vi "Main.vi"(11 "Module Admin":refnum<class "Delacor_lib_QMH_Module Admin.lvclass">) -> ()   [LabVIEW 2025, in "Autofrettage UI.lvlib"]
doc: "This template is based off of the Queued Message Handler design pattern and the Queued Message Handler project template that ships with LabVIEW.\n\nThe main difference is that the queue is private to this module and communication between modules is performed via Broadcast and Request events.\n\nRequest events are wrapped in public API methods and are handled in the Event Handling Loop (EHL) of this VI. Any module can register for Broadcast events sent by this module. The EHL generates messages based on user interface actions.\n\nThe Message Handling Loop (MHL) processes messages generated by the EHL, or by other messages. The messages are string values, so new messages can be added easily to the Message Cases case structure in the MHL. Each message cluster can also provide an optional value for Message Data, which is a variant that can be converted to whatever message-specific data is required.\n_____\nBased on DQMH Project Template 4.0.0.47.\n_____\nBased on DQMH Dev Tools: Project Template 7.1.0.1503."
uses:
  Autofrettage UI.lvlib
  Module Data--cluster.ctl
  <vilib>/Delacor/Delacor QMH/Libraries/Message Queue_class/Delacor_lib_QMH_Message Queue.lvclass
  <vilib>/Delacor/Delacor QMH/Libraries/Message Queue_class/Delacor_lib_QMH_Enqueue Message (Single).vi
  <vilib>/Delacor/Delacor QMH/Libraries/Module Admin_class/Delacor_lib_QMH_Module Admin.lvclass
  Stop Argument--cluster.ctl
  Settings Editor/Settings Editor.lvlib
  Acquisition/Acquisition.lvlib
  Logger/Logger.lvlib
  Settings Editor/Test Meta Data.ctl
panel:
  out "Horizontal Pointer Slide":dbl(slide) scale=0.0..100000.0
  in  "Part Number":string
  in  "Job Number":string
  in  "Operator":string
  in  "ZERO":bool
  out "Numeric":dbl format="%.0f PSI"
  out "Data":waveform(dbl)[](graph)
  in  "Start Logging":bool
  in  "Settings":bool
  in  "Start":bool
  in  "Stop":bool
  out "error out":errorcluster
  out "Status":string
  in  "About":bool
  out "Logger Running?":bool
  out "Settings Editor Running?":bool
  out "Acquisition Running?":bool
  out "version":string
  # "Autofrettage"
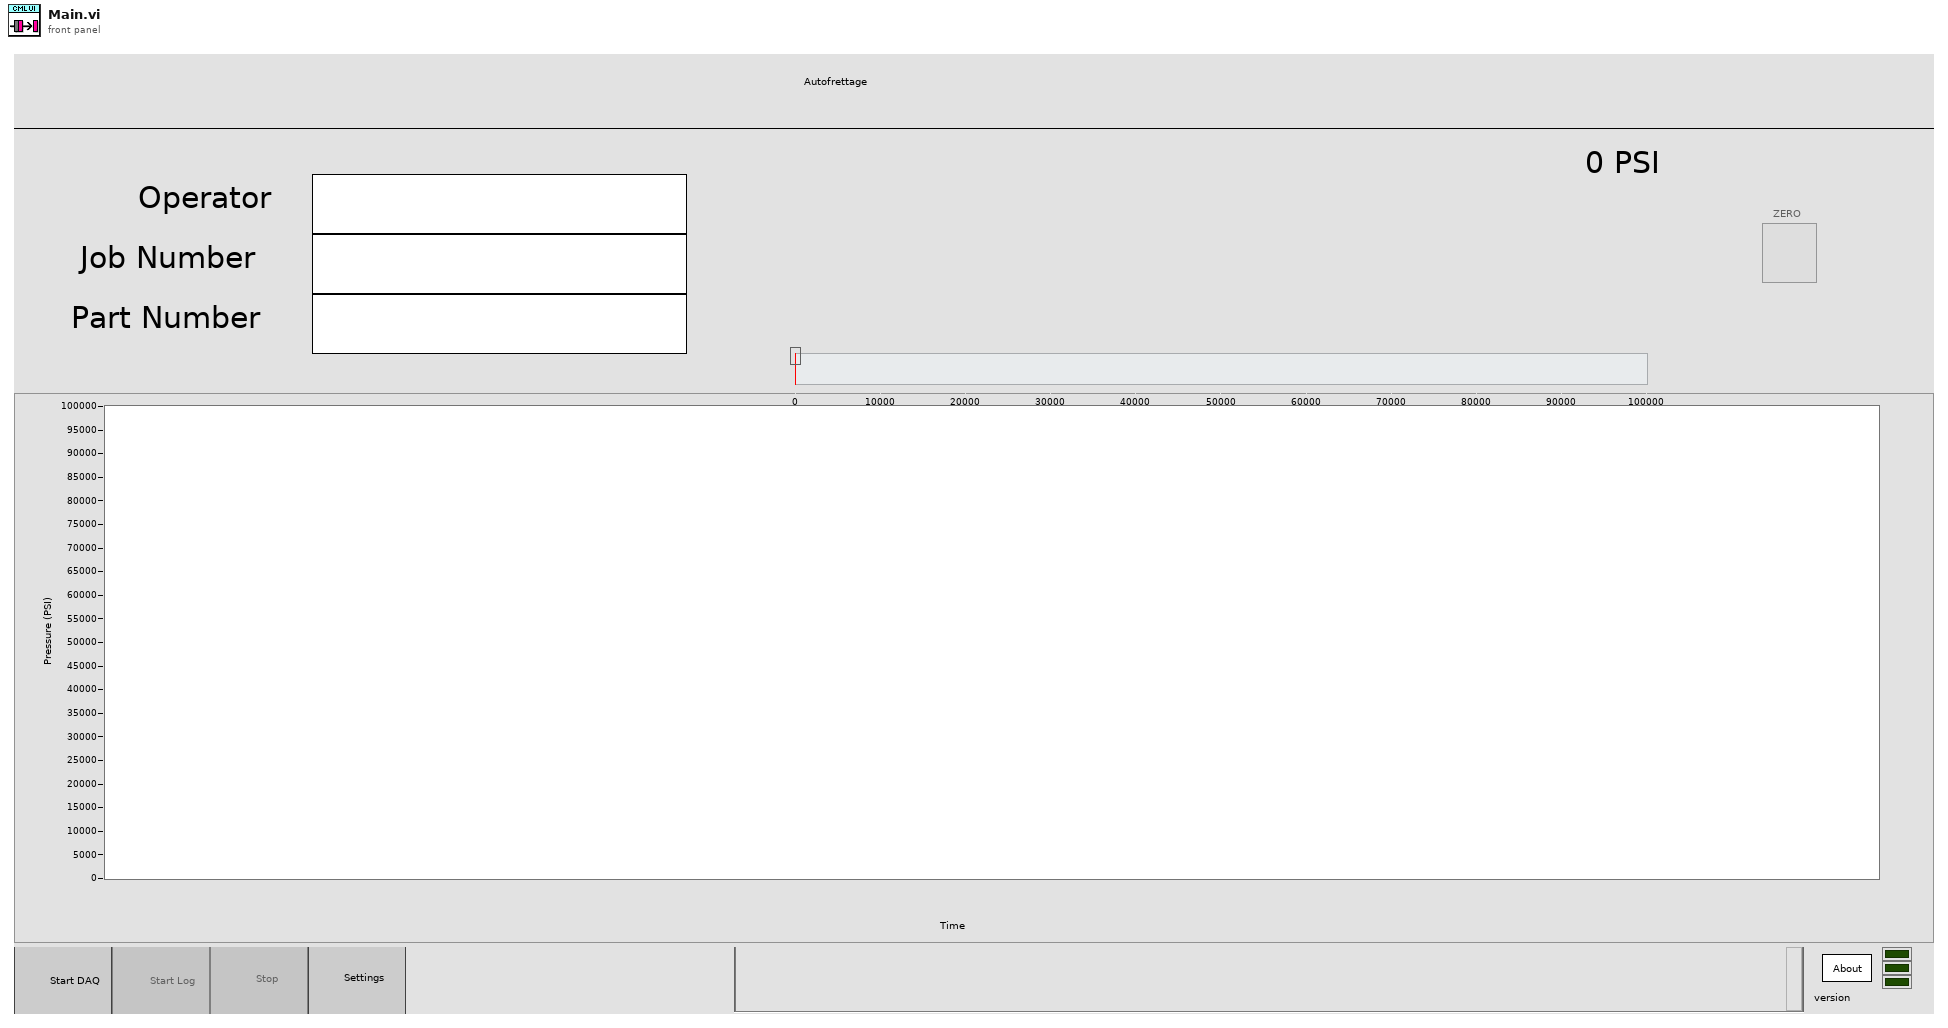
[diagram p1: front panel]
types:
  T1 = typedef "Autofrettage UI.lvlib/Request Events--cluster.ctl" = cluster{"Stop Module":refnum<user-event>, "Show Panel":refnum<user-event>, "Hide Panel":refnum<user-event>, "Get Module Execution Status":refnum<user-event>, "Show Diagram":refnum<user-event>}
  T2 = typedef "Settings Editor.lvlib/Broadcast Events--cluster.ctl" = cluster{"Module Did Init":refnum<user-event>, "Status Updated":refnum<user-event>, "Error Reported":refnum<user-event>, "Module Did Stop":refnum<user-event>, "Update Module Execution Status":refnum<user-event>, "Application Settings Updated":refnum<user-event>}
  T3 = typedef "Acquisition.lvlib/Broadcast Events--cluster.ctl" = cluster{"Module Did Init":refnum<user-event>, "Status Updated":refnum<user-event>, "Error Reported":refnum<user-event>, "Module Did Stop":refnum<user-event>, "Update Module Execution Status":refnum<user-event>, "Acquisition Started":refnum<user-event>, "Acquisition Stopped":refnum<user-event>, "Data Updated":refnum<user-event>, "Tare Updated":refnum<user-event>}
  T4 = typedef "Logger.lvlib/Broadcast Events--cluster.ctl" = cluster{"Module Did Init":refnum<user-event>, "Status Updated":refnum<user-event>, "Error Reported":refnum<user-event>, "Module Did Stop":refnum<user-event>, "Update Module Execution Status":refnum<user-event>, "Logging Stopped":refnum<user-event>, "File Initialized":refnum<user-event>}
  T5 = typedef "Autofrettage UI.lvlib/Module Data--cluster.ctl" = cluster{"Status":string, "Start DAQ Ref":refnum<vi>, "Settings Ref":refnum<vi>, "Stop Ref":refnum<vi>, "Status Ref":refnum<vi>, "Data Ref":refnum<vi>, "Start Logging Ref":refnum<vi>, "Tare Ref":refnum<vi>}
  T6 = enum32{"invalid lock state", "Not Locked", "Locked (No Password)", "Password-protected"}
  T7 = typedef "Autofrettage UI.lvlib/Stop Argument--cluster.ctl" = cluster{"Origin":string, "Exit via Stop Module Req?":bool, "Wait for Module to stop?":bool}
  T8 = enum32{"Invalid", "Standard", "Closed", "Hidden", "Minimized", "Maximized"}
  T9 = typedef "Settings Editor.lvlib/Test Meta Data.ctl" = cluster{"Operator":string, "Job Number":string, "Part Number":string}
  T10 = typedef "Settings Editor.lvlib/Update Application Settings (Reply Payload)--cluster.ctl" = cluster{"Settings":T11, "error":errorcluster}
  T11 = typedef "Settings Editor.lvlib/Settings--cluster.ctl" = cluster{"Log File Base Path":path, "Meta Data":T12, "DAQ Settings":cluster{"physical channel":string, "minimum value":dbl, "maximum value":dbl, "number of samples":i32, "rate":dbl, "custom scale name":string}}
  T12 = typedef "Test Meta Data.ctl" = cluster{"Operator":string, "Job Number":string, "Part Number":string}
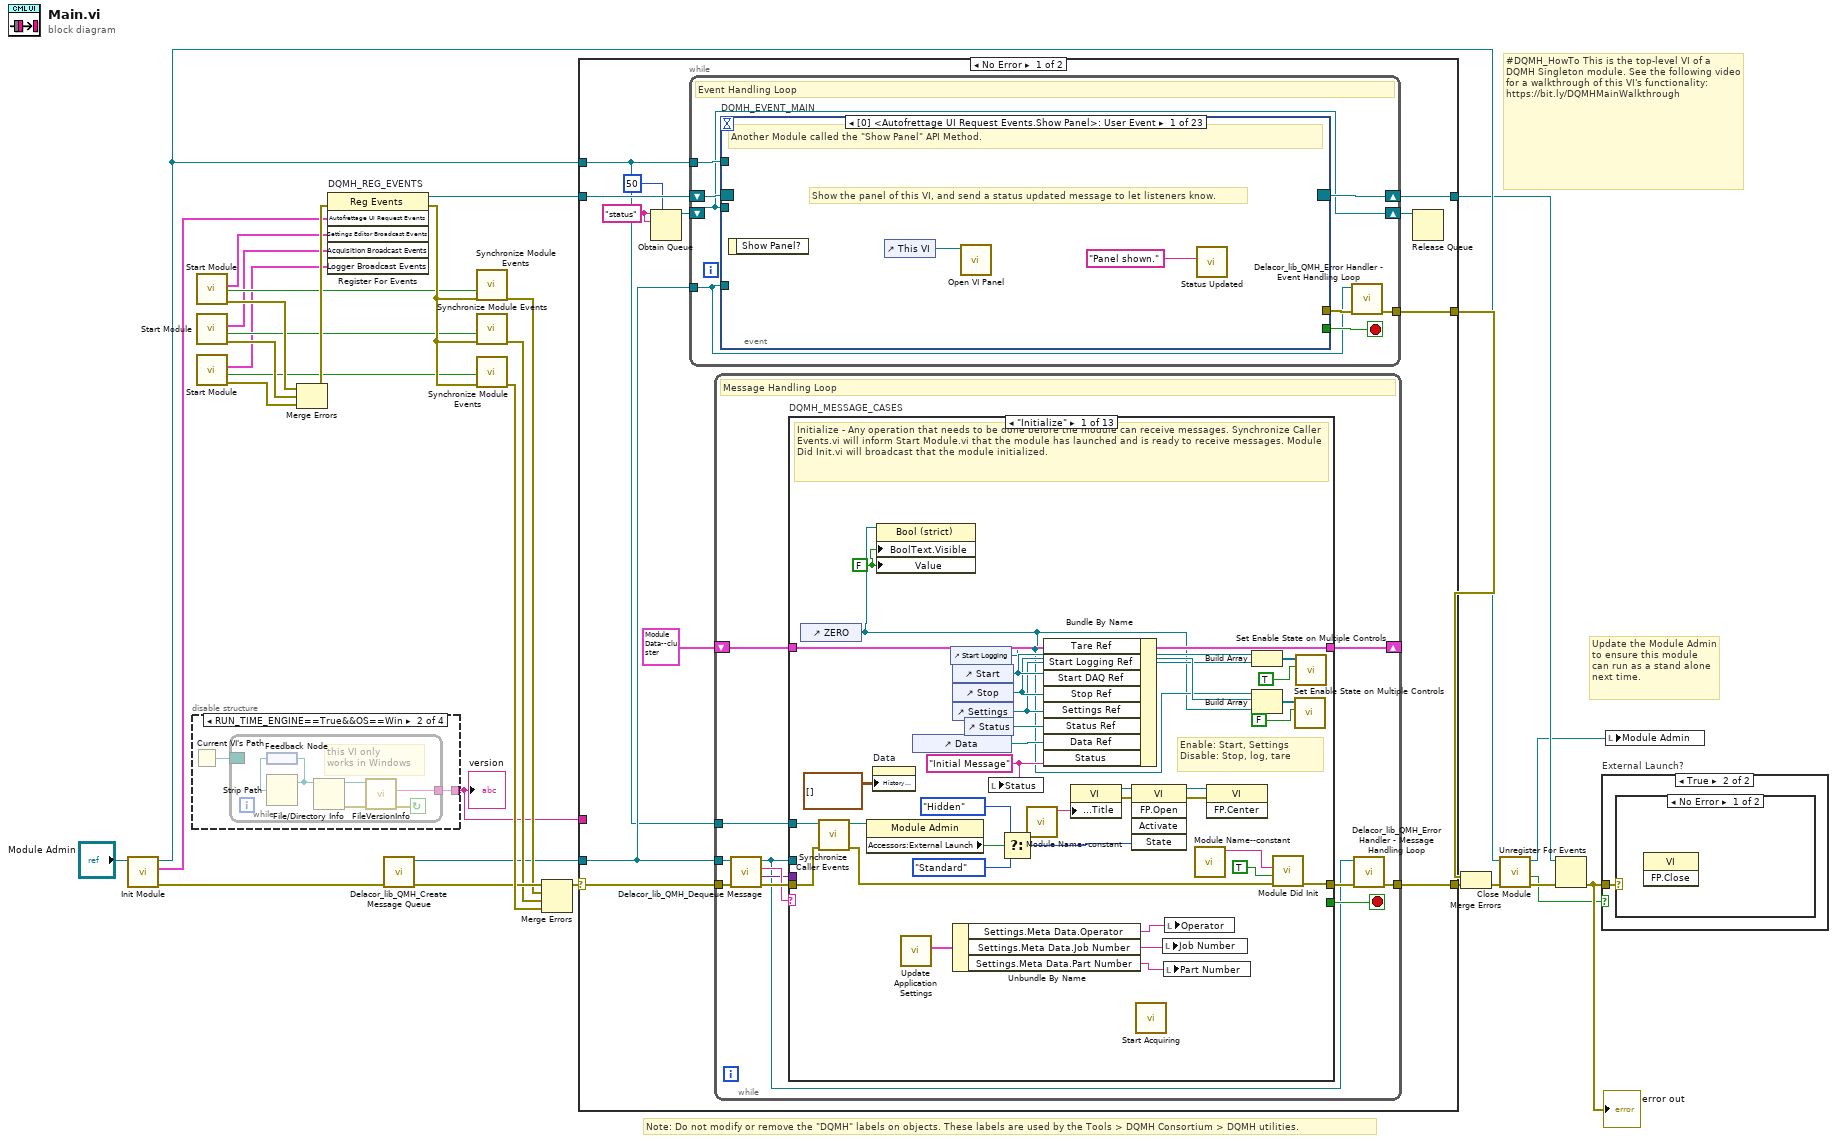
[diagram p0: block diagram]
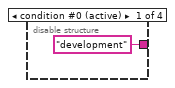
[diagram p2: hidden frame]
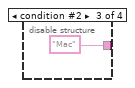
[diagram p3: hidden frame]
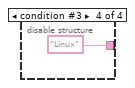
[diagram p4: hidden frame]
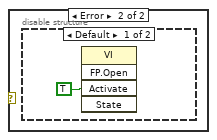
[diagram p6: hidden frame]
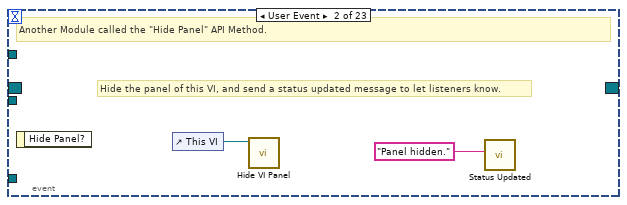
[diagram p8: hidden frame]
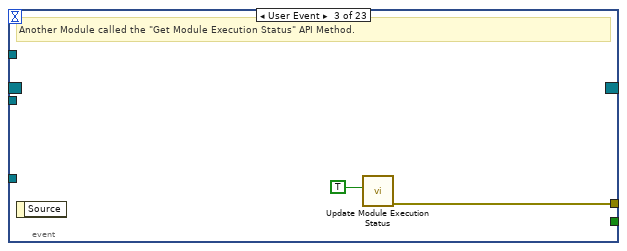
[diagram p9: hidden frame]
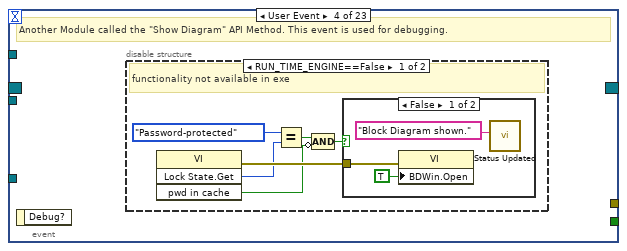
[diagram p10: hidden frame]
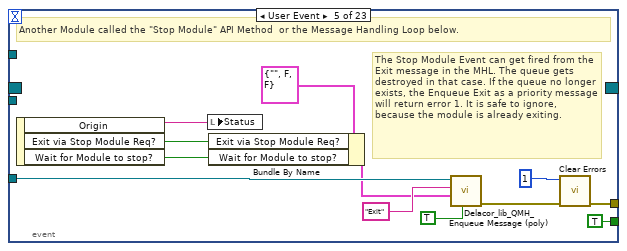
[diagram p13: hidden frame]
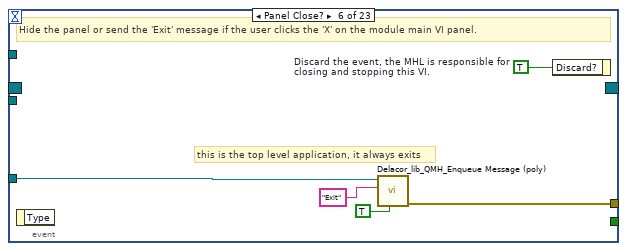
[diagram p14: hidden frame]
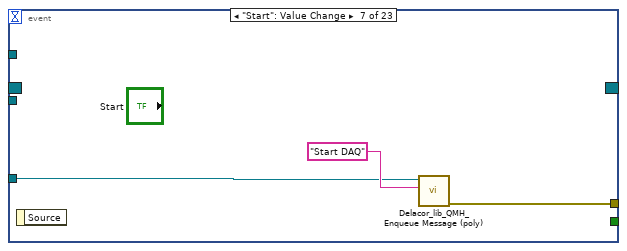
[diagram p15: hidden frame]
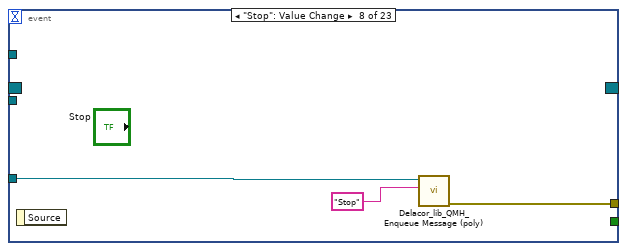
[diagram p16: hidden frame]
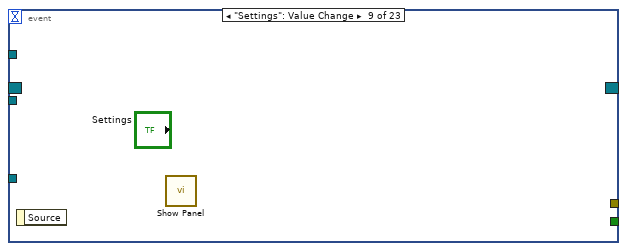
[diagram p17: hidden frame]
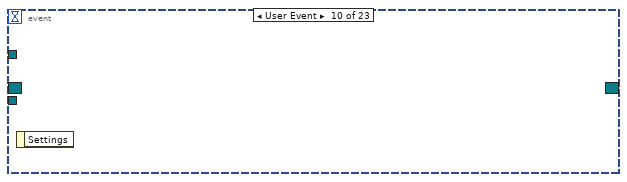
[diagram p18: hidden frame]
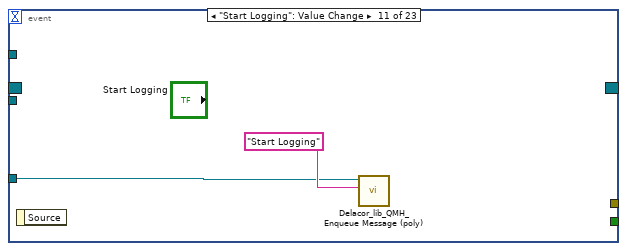
[diagram p19: hidden frame]
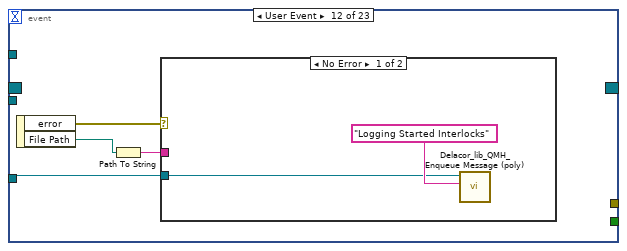
[diagram p20: hidden frame]
diagram:
  # "#DQMH_HowTo This is the top-level VI of a DQMH Singleton module. See the following video for a walkthrough of this VI's functionality: https://bit.ly/DQMHMainWalkthrough"
  # "Note: Do not modify or remove the \"DQMH\" labels on objects. These labels are used by the Tools > DQMH Consortium > DQMH utilities."
  # "Update the Module Admin to ensure this module can run as a stand alone next time."
  n1 = call "Init Module.vi"("Singleton Module Admin in"="Module Admin") -> ("error out"=w29:errorcluster, "Autofrettage UI Request Events"=w12:T1, "Singleton Module Admin out"=w15:refnum<class "Delacor_lib_QMH_Module Admin.lvclass">)  [unwired: 8 in]
  n2 = disable-structure "Conditional Disable Structure" shown="RUN_TIME_ENGINE==True&&OS==Win" {
    disable-tunnel: ["development" w33 "Mac" "Linux"] -> w1
    frame condition #0 (active) {
    }
    frame condition #1 {
      n3 = Current VI's Path() -> (path=w34:path)
      n4 = while {
        border: w34 -> [_]
        tunnel: [w35] -> w33
        stop <- w39 continue-if-true
        # "this VI only \nworks in Windows"
        n5 = feedback #1() -> (w38:path)
        n6 = Strip Path(path=w38) -> (stripped path=w37:path)  [unwired: 1 out]
        n7 = feedback-in #1(w37) -> ()
        n8 = File/Directory Info(path=w37) -> (path out=w36:path, error out=w40:errorcluster)  [unwired: 1 in, 5 out]
        n9 = call <vilib>:"FileVersionInfo.vi"("error in (no error)"=w40, "Application Path in"=w36) -> ("error out"=w39:errorcluster, "File Version Info"=w35:string)  [unwired: 6 in, 2 out]
      }
    }
    frame condition #2 {
    }
    frame condition #3 {
    }
  }
  "version" <- w1
  n10 = call "Start Module.vi"() -> ("error out"=w20:errorcluster, "Wait for Event Sync?"=w7:bool, "Settings Editor Broadcast Events"=w6:T2)  [unwired: 7 in, 2 out]
  n11 = call "Start Module.vi"() -> ("error out"=w19:errorcluster, "Wait for Event Sync?"=w4:bool, "Acquisition Broadcast Events"=w5:T3)  [unwired: 7 in, 2 out]
  n12 = call "Start Module.vi"() -> ("error out"=w18:errorcluster, "Wait for Event Sync?"=w2:bool, "Logger Broadcast Events"=w3:T4)  [unwired: 7 in, 2 out]
  n13 = Merge Errors(w20, w19, w18) -> (w17:errorcluster)
  n14 = register-events "DQMH_REG_EVENTS"(error in=w17, w12, w6, w5, w3) -> (reference out=w13:refnum<event-registration>, error out=w16:errorcluster)  [unwired: 1 in]
  n15 = call <vilib>:"Delacor_lib_QMH_Create Message Queue.vi"("error in"=w29) -> ("error out"=w24:errorcluster, "Message Queue"=w11:refnum<class "Delacor_lib_QMH_Message Queue.lvclass">)  [unwired: 9 in]
  n16 = call "Synchronize Module Events.vi"("error in"=w16, "Wait for Event Sync?"=w7) -> ("error out"=w22:errorcluster)  [unwired: 9 in]
  n17 = call "Synchronize Module Events.vi"("error in"=w16, "Wait for Event Sync?"=w4) -> ("error out"=w21:errorcluster)  [unwired: 9 in]
  n18 = call "Synchronize Module Events.vi"("error in"=w16, "Wait for Event Sync?"=w2) -> ("error out"=w31:errorcluster)  [unwired: 9 in]
  n19 = Merge Errors(w24, w22, w21, w31) -> (w23:errorcluster)
  n20 = case shown="No Error" w23 {
    selector: w23 -> [w52 w315]
    tunnel: [w54 w314] -> w30
    tunnel: [w51 w313] -> w14
    tunnel: w13 -> [w49 w313]
    tunnel: w11 -> [w48 w306]
    tunnel: [w53 _] -> w27
    tunnel: w15 -> [w47 w309]
    tunnel: w1 -> [_ _]
    frame No Error {
      w43 = "status" ("name (unnamed)")
      n21 = Obtain Queue(max queue size (-1, unlimited)=50, name (unnamed)=w43, element data type=w43) -> (queue out=w45:refnum<queue>)  [unwired: 2 in, 2 out]
      n22 = while {
        tunnel: w48 -> [w56]
        shift-right: [w59] -> w51
        shift-left: w49 -> [w60]
        tunnel: [w61] -> w53
        tunnel: w47 -> [w57]
        shift-right: [w55] -> w44
        shift-left: w45 -> [w55]
        stop <- w58 stop-if-true
        # "Event Handling Loop"
        n23 = event "DQMH_EVENT_MAIN" shown="[0] <Autofrettage UI Request Events.Show Panel>: User Event" {
          selector: w60 -> [_ _ _ _ _ _ _ _ _ _ _ _ _ _ w118 _ _ _ _ _ _ _ _]
          dyn-events: [_ _ _ _ _ _ _ _ _ _ _ _ _ _ w118 _ _ _ _ _ _ _ _] -> w59
          timeout: _ -> [_ _ _ _ _ _ _ _ _ _ _ _ _ _ _ _ _ _ _ _ _ _ _]
          tunnel: [_ _ _ _ TRUE ("Discard?") _ _ _ _ _ _ _ _ _ _ _ _ _ _ _ _ _ _] -> w58
          tunnel: w56 -> [_ _ _ _ w85 w92 w95 w98 _ _ w101 w103 _ _ _ _ _ _ w144 w148 _ _ _]
          tunnel: [_ _ w68 _ w88 w94 w97 w100 _ _ _ _ _ _ _ _ _ w139 _ _ _ _ w155] -> w62
          tunnel: w57 -> [_ _ _ _ _ _ _ _ _ _ _ _ _ _ _ _ _ _ _ _ _ _ _]
          tunnel: w55 -> [_ _ _ _ _ _ _ _ _ _ _ _ _ _ _ _ w133 _ _ _ _ _ _]
          event User Event {
            # "Show the panel of this VI, and send a status updated message to let listeners know."
            # "Another Module called the \"Show Panel\" API Method."
            n24 = event-data() -> ()  [unwired: 1 in, 1 out]
            n25 = control-ref of="This VI"() -> (w64:refnum<vi>)
            n26 = call "Open VI Panel.vi"("VI"=w64) -> ()  [unwired: 10 in, 1 out]
            n27 = call "Status Updated.vi"("Status"="Panel shown." ("format string")) -> ()  [unwired: 10 in, 1 out]
          }
          event User Event {
            # "Hide the panel of this VI, and send a status updated message to let listeners know."
            # "Another Module called the \"Hide Panel\" API Method."
            n28 = event-data() -> ()  [unwired: 1 in, 1 out]
            n29 = control-ref of="This VI"() -> (w66:refnum<vi>)
            n30 = call "Hide VI Panel.vi"("VI"=w66) -> ()  [unwired: 10 in, 1 out]
            n31 = call "Status Updated.vi"("Status"="Panel hidden." ("format string")) -> ()  [unwired: 10 in, 1 out]
          }
          event User Event {
            # "Another Module called the \"Get Module Execution Status\" API Method."
            n32 = event-data() -> ()  [unwired: 1 in, 1 out]
            n33 = call "Update Module Execution Status.vi"("Running?"=TRUE) -> ("error out"=w68:errorcluster)  [unwired: 10 in]
          }
          event User Event {
            # "Another Module called the \"Show Diagram\" API Method. This event is used for debugging."
            n34 = event-data() -> ()  [unwired: 1 in, 1 out]
            n35 = disable-structure shown="RUN_TIME_ENGINE==False" {
              frame condition #0 (active) {
                # "functionality not available in exe"
                n36 = invoke on="Invoke Node" class="VI" method="Lock State.Get"() -> (error out=w74:errorcluster, "Get Lock State"=w73:T6, "pwd in cache"=w70:bool)  [unwired: 4 in, 1 out]
                n37 = Equal?(x=T6."Password-protected", y=w73) -> (x = y?=w71:bool)
                n38 = Compound Arithmetic op=AND(w71, invert w70) -> (w69:bool)
                n39 = case shown="False" w69 {
                  tunnel: w74 -> [w77 _]
                  frame False {
                    n40 = property on="Property Node" class="VI"(error in=w77, "BDWin.Open"=TRUE ("Block Diagram Window:Open")) -> ()  [unwired: 1 in, 2 out]
                    n41 = call "Status Updated.vi"("Status"="Block Diagram shown." ("format string")) -> ()  [unwired: 10 in, 1 out]
                  }
                  frame True {
                    # "Password-protected VI, and the password is not in the cache. Do not show the diagram."
                  }
                }
              }
              frame condition #1 {
              }
            }
          }
          event User Event {
            # "The Stop Module Event can get fired from the Exit message in the MHL. The queue gets destroyed in that case. If the queue no longer exists, the Enqueue Exit as a priority message will return error 1. It is safe to ignore, because the module is already exiting."
            # "Another Module called the \"Stop Module\" API Method  or the Message Handling Loop below."
            n42 = event-data() -> ("Origin"=w84:string, "Exit via Stop Module Req?"=w80:bool, "Wait for Module to stop?"=w79:bool)  [unwired: 1 in]
            n43 = local write "Status"(w84) -> ()
            n44 = Bundle By Name(cluster=T7 {"Origin"="", "Exit via Stop Module Req?"=FALSE, "Wait for Module to stop?"=FALSE} ("Stop Argument"), "Exit via Stop Module Req?"=w80, "Wait for Module to stop?"=w79) -> (w78:T7)
            n45 = call-poly <vilib>:"Delacor_lib_QMH_Enqueue Message (poly).vi"("Priority Message? (F)"=TRUE, "Message Data"=w78, "Message"="Exit", "Message Queue in"=w85) -> ("error out"=w89:errorcluster)  [unwired: 6 in, 1 out]
            n46 = call <vilib>:"Clear Errors.vi"("error in (no error)"=w89, "specific error code to clear (0: all)"=1) -> ("error out"=w88:errorcluster)  [unwired: 4 in, 1 out]
          }
          event Panel Close? {
            w93 = TRUE  # Discard the event, the MHL is responsible for closing and stopping this VI.
            # "this is the top level application, it always exits"
            # "Hide the panel or send the 'Exit' message if the user clicks the 'X' on the module main VI panel."
            n47 = event-data() -> ()  [unwired: 1 in, 1 out]
            n48 = call-poly <vilib>:"Delacor_lib_QMH_Enqueue Message (poly).vi"("Priority Message? (F)"=TRUE, "Message"="Exit", "Message Queue in"=w92) -> ("error out"=w94:errorcluster)  [unwired: 7 in, 1 out]
            n49 = event-data ("Event Filter Node")("Discard?"=w93) -> ()  [unwired: 1 in, 1 out]
          }
          event "Start": Value Change {
            n50 = event-data() -> ()  [unwired: 1 in, 1 out]
            n51 = call-poly <vilib>:"Delacor_lib_QMH_Enqueue Message (poly).vi"("Message"="Start DAQ", "Message Queue in"=w95) -> ("error out"=w97:errorcluster)  [unwired: 8 in, 1 out]
          }
          event "Stop": Value Change {
            n52 = event-data() -> ()  [unwired: 1 in, 1 out]
            n53 = call-poly <vilib>:"Delacor_lib_QMH_Enqueue Message (poly).vi"("Message"="Stop", "Message Queue in"=w98) -> ("error out"=w100:errorcluster)  [unwired: 8 in, 1 out]
          }
          event "Settings": Value Change {
            n54 = event-data() -> ()  [unwired: 1 in, 1 out]
            n55 = call "Show Panel.vi"() -> ()  [unwired: 11 in, 1 out]
          }
          event User Event {
            n56 = event-data() -> ()  [unwired: 1 in, 1 out]
          }
          event "Start Logging": Value Change {
            n57 = event-data() -> ()  [unwired: 1 in, 1 out]
            n58 = call-poly <vilib>:"Delacor_lib_QMH_Enqueue Message (poly).vi"("Message"="Start Logging", "Message Queue in"=w101) -> ()  [unwired: 8 in, 2 out]
          }
          event User Event {
            n59 = event-data() -> ("error"=w106:errorcluster, "File Path"=w105:path)  [unwired: 1 in]
            n60 = Path To String(path=w105) -> (string=w104:string)
            n61 = case shown="No Error" w106 {
              tunnel: w104 -> [_ _]
              tunnel: w103 -> [w107 _]
              frame No Error {
                n62 = call-poly <vilib>:"Delacor_lib_QMH_Enqueue Message (poly).vi"("Message"="Logging Started Interlocks", "Message Queue in"=w107) -> ()  [unwired: 8 in, 2 out]
              }
              frame Error {
              }
            }
          }
          event "ZERO": Value Change {
            n63 = event-data() -> ()  [unwired: 1 in, 1 out]
            n64 = call "Set Tare.vi"("Tare"="ZERO") -> ()  [unwired: 10 in, 1 out]
          }
          event User Event {
            w111 = TRUE ("Settings Editor Running?")
            n65 = event-data() -> ()  [unwired: 1 in, 1 out]
            n66 = local read "Acquisition Running?"() -> (w113:bool)
            n67 = local read "Logger Running?"() -> (w112:bool)
            n68 = call "Is UI Ready.vi"("Logger Running?"=w112, "Acquisition Running?"=w113, "Settings Editor Running?"=w111) -> ("Status"=w110:string)  [unwired: 8 in]
            n69 = local write "Status"(w110) -> ()
            "Settings Editor Running?" <- w111
          }
          event User Event {
            w116 = TRUE ("Acquisition Running?")
            n70 = event-data() -> ()  [unwired: 1 in, 1 out]
            n71 = local read "Settings Editor Running?"() -> (w115:bool)
            n72 = local read "Logger Running?"() -> (w114:bool)
            n73 = call "Is UI Ready.vi"("Logger Running?"=w114, "Acquisition Running?"=w116, "Settings Editor Running?"=w115) -> ("Status"=w117:string)  [unwired: 8 in]
            n74 = local write "Status"(w117) -> ()
            "Acquisition Running?" <- w116
          }
          event User Event {
            w121 = TRUE ("Logger Running?")
            n75 = event-data() -> ()  [unwired: 1 in, 1 out]
            n76 = local read "Settings Editor Running?"() -> (w120:bool)
            n77 = local read "Acquisition Running?"() -> (w119:bool)
            n78 = call "Is UI Ready.vi"("Logger Running?"=w121, "Acquisition Running?"=w119, "Settings Editor Running?"=w120) -> ("Status"=w122:string)  [unwired: 8 in]
            n79 = local write "Status"(w122) -> ()
            "Logger Running?" <- w121
          }
          event User Event {
            n80 = event-data() -> ("Status"=w125:string)  [unwired: 1 in]
            n81 = Format Date/Time String(time format string (%c)="%H:%M:%S%3u") -> (date/time string=w127:string)  [unwired: 2 in]
            n82 = Format Into String(format string="%s: %s", w127, w125) -> (resulting string=w124:string)  [unwired: 2 in, 1 out]
            n83 = Lossy Enqueue Element(queue=w133, element=w124) -> (queue out=w132:refnum<queue>)  [unwired: 1 in, 3 out]
            n84 = Get Queue Status(queue=w132, return elements? (F)=TRUE) -> (elements=w130:string[])  [unwired: 1 in, 7 out]
            n85 = Reverse 1D Array(array=w130) -> (reversed array=w129:string[])
            n86 = for {
              tunnel: w129 -> [w136] mode=indexing
              tunnel: [w134] -> w128 mode=concatenating
              n87 = Concatenate Strings(w136, "\r\n") -> (w134:string)
            }
            "Status" <- w128
            n88 = call "Status Updated.vi"("Status"=w128) -> ()  [unwired: 10 in, 1 out]
          }
          event User Event {
            n89 = event-data() -> ("Error"=w139:errorcluster, "Module Name"=w141:string)  [unwired: 1 in]
            n90 = Unbundle By Name(w139) -> ("code"=w142:i32)
            n91 = Format Into String(format string="Error %d at %s", w142, w141) -> (resulting string=w138:string)  [unwired: 2 in, 1 out]
            n92 = Bundle By Name(cluster=w139, "source"=w138) -> (w137:errorcluster)
            n93 = call <vilib>:"Simple Error Handler.vi"("error in (no error)"=w137) -> ()  [unwired: 4 in, 5 out]
          }
          event User Event {
            n94 = event-data() -> ("Success"=w143:bool)  [unwired: 1 in]
            n95 = case shown="True" w143 {
              tunnel: w144 -> [_ w146]
              frame False {
              }
              frame True {
                n96 = call-poly <vilib>:"Delacor_lib_QMH_Enqueue Message (poly).vi"("Message"="Acquisition Started Interlocks", "Message Queue in"=w146) -> ()  [unwired: 8 in, 2 out]
              }
            }
          }
          event User Event {
            n97 = event-data() -> ()  [unwired: 1 in, 1 out]
            n98 = call-poly <vilib>:"Delacor_lib_QMH_Enqueue Message (poly).vi"("Message"="Acquisition Stopped Interlocks", "Message Queue in"=w148) -> ()  [unwired: 8 in, 2 out]
          }
          event User Event {
            n99 = event-data() -> ("Numeric"=→"Numeric" →"Horizontal Pointer Slide":dbl, "Graph Data"=→"Data":waveform(dbl)[])  [unwired: 1 in]
          }
          event User Event {
            n100 = event-data() -> ("Tare Offset"=w154:dbl)  [unwired: 1 in]
            n101 = Not Equal To 0?(x=w154) -> (x != 0?=w151:bool)
            n102 = Format Into String(format string="%d", w154) -> (resulting string=w152:string)  [unwired: 2 in, 1 out]
            n103 = property on="ZERO" class="Bool (strict)"("Value"=w151, "BoolText.Visible"=w151, "BoolText.Text"=w152) -> ()  [unwired: 2 in, 2 out]
          }
          event "About": Value Change {
            # "Display the About DQMH box"
            n104 = event-data() -> ()  [unwired: 1 in, 1 out]
            n105 = call <vilib>:"DQMH_About Box.vi"() -> ("error out"=w155:errorcluster)  [unwired: 11 in]
          }
        }
        n106 = call-dynamic "Delacor_lib_QMH_Error Handler - Event Handling Loop.vi"("error in"=w62, "Message Queue in"=w56) -> ("dup error in"=w61:errorcluster)  [unwired: 8 in, 1 out]
      }
      n107 = while {
        tunnel: w48 -> [w158]
        shift-right: [w162] -> _
        shift-left: T5 {"Status"="", "Start DAQ Ref"=refnum, "Settings Ref"=refnum, "Stop Ref"=refnum, "Status Ref"=refnum, "Data Ref"=refnum, "Start Logging Ref"=refnum, "Tare Ref"=refnum} ("Data Cluster") -> [w163]
        tunnel: w52 -> [w166]
        tunnel: [w164] -> w54
        tunnel: w47 -> [w156]
        stop <- w161 stop-if-true
        # "Message Handling Loop"
        n108 = call-dynamic "Delacor_lib_QMH_Dequeue Message.vi"("error in"=w166, "Message Queue in"=w158) -> ("error out"=w165:errorcluster, "Message Data"=w159:variant, "Message"=w160:string, "Message Queue out"=w157:refnum<class "Delacor_lib_QMH_Message Queue.lvclass">)  [unwired: 6 in]
        n109 = case "DQMH_MESSAGE_CASES" shown="\"Initialize\"" w160 {
          selector: w160 -> [_ _ _ _ _ _ _ _ _ _ _ _ w301]
          tunnel: w157 -> [_ _ _ _ _ _ _ _ _ _ w260 w285 _]
          tunnel: w165 -> [w201 w205 w206 w215 w231 w234 w247 w252 w255 w257 w268 w293 w304]
          tunnel: [w199 w205 w208 w216 w231 w233 w247 w252 w254 w257 w264 w286 w305] -> w167
          tunnel: w163 -> [w190 w204 w207 w217 w223 w232 w239 w249 w253 w256 w262 w284 w302]
          tunnel: [w182 w204 w207 w217 w223 w232 w239 w249 w253 w256 w262 w284 w302] -> w162
          tunnel: [_ _ _ _ _ _ _ _ _ _ _ w283 _] -> w161
          tunnel: w159 -> [_ _ _ _ _ _ _ _ _ _ w261 w282 _]
          tunnel: w156 -> [w191 _ _ _ _ _ _ _ _ _ w259 w277 _]
          frame "Initialize" {
            w169 = FALSE ("Value")
            w185 = "Initial Message" ("Initial Message")
            # "Enable: Start, Settings\nDisable: Stop, log, tare"
            # "Initialize - Any operation that needs to be done before the module can receive messages. Synchronize Caller Events.vi will inform Start Module.vi that the module has launched and is ready to receive messages. Module Did Init.vi will broadcast that the module initialized."
            n110 = control-ref of="ZERO"() -> (w168:refnum<vi>)
            n111 = call "Synchronize Caller Events.vi"("error in"=w201, "Singleton Module Admin in"=w191) -> ("error out"=w200:errorcluster, "Singleton Module Admin out"=w187:refnum<class "Delacor_lib_QMH_Module Admin.lvclass">)  [unwired: 8 in]
            n112 = property on="Property Node" class="Module Admin"(reference=w187) -> ("Accessors:External Launch"=w195:bool)  [unwired: 1 in, 2 out]
            n113 = property on="Data" class="WFChart (strict)"("History Data"=waveform(dbl)[][] []) -> ()  [unwired: 2 in, 2 out]
            n114 = property class="Bool (strict)"(reference=w168, "BoolText.Visible"=w169, "Value"=w169) -> ()  [unwired: 1 in, 2 out]
            n115 = call "Update Application Settings.vi"() -> ("Reply Payload"=w170:T10)  [unwired: 9 in, 2 out]
            n116 = control-ref of="Data"() -> (w183:refnum<vi>)
            n117 = control-ref of="Start Logging"() -> (w174:refnum<vi>)
            n118 = control-ref of="Start"() -> (w177:refnum<vi>)
            n119 = control-ref of="Stop"() -> (w176:refnum<vi>)
            n120 = control-ref of="Settings"() -> (w175:refnum<vi>)
            n121 = Unbundle By Name(w170) -> ("Settings.Meta Data.Operator"=w171:string, "Settings.Meta Data.Job Number"=w172:string, "Settings.Meta Data.Part Number"=w173:string)
            n122 = control-ref of="Status"() -> (w184:refnum<vi>)
            n123 = local write "Status"(w185) -> ()
            n124 = Select(t=T8."Hidden" ("State"), s=w195, f=T8."Standard" ("State")) -> (s? t:f=w192:T8)
            n125 = call "Module Name--constant.vi"() -> ("Module Name"=w198:string)  [unwired: 11 in]
            n126 = Bundle By Name(cluster=w190, "Tare Ref"=w168, "Start Logging Ref"=w174, "Start DAQ Ref"=w177, "Stop Ref"=w176, "Settings Ref"=w175, "Status Ref"=w184, "Data Ref"=w183, "Status"=w185) -> (w182:T5)
            n127 = property on="Property Node" class="VI"("Front Panel.Title"=w198) -> (reference out=w197:refnum<vi>, error out=w203:errorcluster)  [unwired: 2 in]
            n128 = invoke on="Invoke Node" class="VI" method="FP.Open"(reference=w197, error in=w203, "State"=w192) -> (reference out=w196:refnum<vi>, error out=w202:errorcluster)  [unwired: 2 in, 3 out]
            n129 = call "Start Acquiring.vi"() -> ()  [unwired: 9 in, 3 out]
            n130 = local write "Job Number"(w172) -> ()
            n131 = local write "Part Number"(w173) -> ()
            n132 = local write "Operator"(w171) -> ()
            n133 = call "Module Name--constant.vi"() -> ("Module Name"=w188:string)  [unwired: 11 in]
            n134 = invoke on="Invoke Node" class="VI" method="FP.Center"(reference=w196, error in=w202) -> ()  [unwired: 1 in, 3 out]
            n135 = Build Array(w177, w175) -> (w181:refnum<vi>[])
            n136 = Build Array(w174, w176, w168) -> (w179:refnum<vi>[])
            n137 = call "Module Did Init.vi"("error in"=w200, "Initialized?"=TRUE, "Origin"=w188) -> ("error out"=w199:errorcluster)  [unwired: 8 in]
            n138 = call "Set Enable State on Multiple Controls.vi"("Enable?"=FALSE, "Controls"=w179) -> ()  [unwired: 10 in]
            n139 = call "Set Enable State on Multiple Controls.vi"("Enable?"=TRUE, "Controls"=w181) -> ()  [unwired: 10 in]
          }
          frame "---Module Specific---" {
            # "Separator -- The following cases handle messages specific to this Module."
          }
          frame "Start DAQ" {
            # "End user pressed Start button. Need to request for Acquisition to start acquiring and for Logger to start logging."
            n140 = call "Start Acquiring.vi"("error in"=w206) -> ("error out"=w208:errorcluster)  [unwired: 8 in, 2 out]
          }
          frame "Start Logging" {
            # "End user pressed Start button. Need to request for Acquisition to start acquiring and for Logger to start logging."
            n141 = Bundle By Name(cluster=T9 {"Operator"="", "Job Number"="", "Part Number"=""} ("Test Meta Data"), "Operator"="Operator", "Job Number"="Job Number", "Part Number"="Part Number") -> (w212:T9)
            n142 = call "Save Test Meta Data.vi"("error in"=w215, "Test Meta Data"=w212) -> ("error out"=w214:errorcluster)  [unwired: 8 in, 1 out]
            n143 = case shown="No Error" w214 {
              selector: w214 -> [w218 w220]
              tunnel: [w219 w220] -> w216
              frame No Error {
                n144 = call "Initialize File.vi"("error in"=w218) -> ("error out"=w219:errorcluster)  [unwired: 8 in, 2 out]
              }
              frame Error {
              }
            }
          }
          frame "Acquisition Started Interlocks" {
            # "Enable: Stop\nDisable: Start, Settings"
            n145 = Unbundle By Name(w223) -> ("Tare Ref"=w221:refnum<vi>, "Start Logging Ref"=w222:refnum<vi>, "Stop Ref"=w230:refnum<vi>, "Start DAQ Ref"=w225:refnum<vi>, "Settings Ref"=w224:refnum<vi>)
            n146 = Build Array(w225, w224) -> (w226:refnum<vi>[])
            n147 = Build Array(w221, w230, w222) -> (w229:refnum<vi>[])
            n148 = call "Set Enable State on Multiple Controls.vi"("Enable?"=FALSE, "Controls"=w226) -> ()  [unwired: 10 in]
            n149 = call "Set Enable State on Multiple Controls.vi"("Enable?"=TRUE, "Controls"=w229) -> ()  [unwired: 10 in]
          }
          frame "Stop" {
            # "End user pressed Stop button. Need to request for Acquisition to stop acquiring and for Logger to stop logging."
            n150 = call "Stop Acquiring.vi"("error in"=w234) -> ("error out"=w235:errorcluster)  [unwired: 10 in]
            n151 = call "Stop Logging.vi"("error in"=w235) -> ("error out"=w233:errorcluster)  [unwired: 10 in]
          }
          frame "Acquisition Stopped Interlocks" {
            w237 = FALSE ("Value")
            # "Enable: Start, Settings\nDisable: Stop"
            n152 = Unbundle By Name(w239) -> ("Tare Ref"=w236:refnum<vi>, "Start Logging Ref"=w238:refnum<vi>, "Stop Ref"=w244:refnum<vi>, "Start DAQ Ref"=w243:refnum<vi>, "Settings Ref"=w242:refnum<vi>)
            n153 = Build Array(w243, w242) -> (w241:refnum<vi>[])
            n154 = Build Array(w236, w238, w244) -> (w246:refnum<vi>[])
            n155 = property class="Bool (strict)"(reference=w236, "BoolText.Visible"=w237, "Value"=w237) -> ()  [unwired: 1 in, 2 out]
            n156 = call "Set Enable State on Multiple Controls.vi"("Enable?"=TRUE, "Controls"=w241) -> ()  [unwired: 10 in]
            n157 = call "Set Enable State on Multiple Controls.vi"("Enable?"=FALSE, "Controls"=w246) -> ()  [unwired: 10 in]
          }
          frame "Logging Started Interlocks" {
            # "Enable: Start, Settings\nDisable: Stop"
            n158 = Unbundle By Name(w249) -> ("Start Logging Ref"=w248:refnum<vi>)
            n159 = Build Array(w248) -> (w251:refnum<vi>[])
            n160 = call "Set Enable State on Multiple Controls.vi"("Enable?"=FALSE, "Controls"=w251) -> ()  [unwired: 10 in]
          }
          frame "---Copy This Frame---" {
            # "Duplicate this frame when creating new messages.  Change this comment in the duplicated frame to describe this message."
            n161 = Merge Errors(w255) -> (w254:errorcluster)
          }
          frame "---Exit and Error Handling---" {
            # "Separator - The following cases handle errors and exit messages."
          }
          frame "Error" {
            # "Error - Check the error message data and respond accordingly. This message is sent by the \"Error Handler\" VIs at the end of each loop in this application."
            n162 = property on="Property Node" class="Module Admin"(reference=w259) -> ("Accessors:External Launch"=w258:bool)  [unwired: 1 in, 2 out]
            n163 = Variant To Data(error in=w268, type=errorcluster {"status"=FALSE, "code"=0, "source"=""} ("error constant"), Variant=w261) -> (data=w263:errorcluster, error out=w266:errorcluster)
            n164 = local write "error out"(w263) -> ()
            n165 = call "Error Reported.vi"("Error"=w263) -> ()  [unwired: 10 in, 1 out]
            n166 = case shown="False" w258 {
              tunnel: [w273 _] -> w265
              tunnel: w260 -> [w271 _]
              tunnel: w263 -> [w272 _]
              frame False {
                n167 = disable-structure shown="Default" {
                  disable-tunnel: w272 -> [w274 _]
                  frame condition #0 (active) {
                    # "If the module is running standalone, then pop up an error dialog and call the \"Exit\" message."
                    n168 = call <vilib>:"Simple Error Handler.vi"("error in (no error)"=w274) -> ()  [unwired: 4 in, 5 out]
                  }
                  frame condition #1 {
                    # "To prevent the Simple Error Handler VI from being loaded (e.g. when deploying to a Real-Time target), add the Conditional Disable Symbol \"DQMH_Disable_SEH\" to your project and set it to TRUE."
                  }
                }
                n169 = call-poly <vilib>:"Delacor_lib_QMH_Enqueue Message (poly).vi"("Priority Message? (F)"=TRUE, "Message"="Exit", "Message Queue in"=w271) -> ("error out"=w273:errorcluster)  [unwired: 7 in, 1 out]
              }
              frame True {
                # "If the module was launched externally, calling the Error Reported broadcast VI is the only action performed by the \"Error\" message. The module's caller can then process the error appropriately."
              }
            }
            n170 = Merge Errors(w266, w265) -> (w264:errorcluster)
          }
          frame "Exit" {
            w276 = TRUE ("Wait for Module to Stop? (F)")
            w283 = TRUE  # Stop the VI
            # "DAQ and LOG modules use the settings editor. CML UI module waits for both modules to completely stop before stopping the settings editor."
            # "Release the message queue reference"
            # "Exit - Exit the application."
            n171 = Variant To Data(error in=w293, type=T7 {"Origin"="", "Exit via Stop Module Req?"=FALSE, "Wait for Module to stop?"=FALSE} ("Stop Argument"), Variant=w282) -> (data=w279:T7, error out=w290:errorcluster)
            n172 = call <vilib>:"Clear Errors.vi"("error in (no error)"=w290, "specific error code to clear (0: all)"=91 ("91: not all Exit messages will have an argument")) -> ("error out"=w292:errorcluster)  [unwired: 4 in, 1 out]
            n173 = control-ref of="This VI"() -> (w278:refnum<vi>)
            n174 = call "Module Name--constant.vi"() -> ("Module Name"=w275:string)  [unwired: 11 in]
            n175 = call "Handle Exit.vi"("Stop Argument"=w279, "Admin in"=w277, "VI reference"=w278) -> ("error out"=w289:errorcluster)  [unwired: 7 in, 1 out]
            n176 = call "Stop Module.vi"("Wait for Module to Stop? (F)"=w276, "Origin"=w275) -> ("error out"=w288:errorcluster)  [unwired: 9 in]
            n177 = call "Stop Module.vi"("Wait for Module to Stop? (F)"=w276, "Origin"=w275) -> ("error out"=w287:errorcluster)  [unwired: 9 in]
            n178 = call-dynamic "Delacor_lib_QMH_Release Message Queue.vi"("error in"=w292, "Message Queue"=w285) -> ("error out"=w291:errorcluster)  [unwired: 9 in]
            n179 = Merge Errors(w288, w287) -> (w294:errorcluster)
            n180 = Merge Errors(w291, w289) -> (w286:errorcluster)
            n181 = call <vilib>:"Clear Errors.vi"("error in (no error)"=w294) -> ("error out"=w295:errorcluster)  [unwired: 5 in, 1 out]
            n182 = call "Error Reported.vi"("Error"=w286) -> ()  [unwired: 10 in, 1 out]
            n183 = call "Stop Module.vi"("error in"=w295, "Wait for Module to Stop? (F)"=w276, "Origin"=w275) -> ()  [unwired: 8 in, 1 out]
          }
          frame Default {
            # "'Default' case only runs if there is a message that isn't defined in any of the other cases.  Output a programming error."
            n184 = call "Module Name--constant.vi"() -> ("Module Name"=w300:string)  [unwired: 11 in]
            n185 = Format Into String(format string="The invalid message string \"%s\" was received in the Message Handling Loop for module \"%s\".", w301, w300) -> (resulting string=w298:string)  [unwired: 2 in, 1 out]
            n186 = call <vilib>:"Error Cluster From Error Code.vi"("show call chain? (False)"=TRUE, "error message (\"\")"=w298, "error code (0)"=1) -> ("error out"=w303:errorcluster)  [unwired: 6 in]
            n187 = Merge Errors(w304, w303) -> (w305:errorcluster)
          }
        }
        n188 = call-dynamic "Delacor_lib_QMH_Error Handler - Message Handling Loop.vi"("error in"=w167, "Message Queue in"=w157) -> ("dup error in"=w164:errorcluster)  [unwired: 8 in, 1 out]
      }
      n189 = Release Queue(queue=w44) -> ()  [unwired: 2 in, 3 out]
    }
    frame Error {
      w308 = TRUE ("Wait for Module to Stop? (F)")
      # "Synchronize Caller Events.vi will inform Start Module.vi that the module has launched and will let the code calling Start Module.vi register for broadcasts and would permit the caller receive the broadcast that an error occurred at launch time."
      n190 = call-dynamic "Delacor_lib_QMH_Release Message Queue.vi"("error in"=w315, "Message Queue"=w306) -> ("error out"=w314:errorcluster)  [unwired: 9 in]
      n191 = call "Synchronize Caller Events.vi"("Singleton Module Admin in"=w309) -> ("error out"=w316:errorcluster)  [unwired: 9 in, 1 out]
      n192 = call "Module Name--constant.vi"() -> ("Module Name"=w312:string)  [unwired: 11 in]
      n193 = call "Module Name--constant.vi"() -> ("Module Name"=w307:string)  [unwired: 11 in]
      n194 = call "Stop Module.vi"("Wait for Module to Stop? (F)"=w308, "Origin"=w307) -> ()  [unwired: 9 in, 1 out]
      n195 = call "Stop Module.vi"("Wait for Module to Stop? (F)"=w308, "Origin"=w307) -> ()  [unwired: 9 in, 1 out]
      n196 = call "Stop Module.vi"("Wait for Module to Stop? (F)"=w308, "Origin"=w307) -> ()  [unwired: 9 in, 1 out]
      n197 = Format Into String(format string="An error occurred during initialization. %s is no longer running.", w312) -> (resulting string=w310:string)  [unwired: 2 in, 1 out]
      n198 = Merge Errors(w314, w316) -> (w317:errorcluster)
      n199 = call "Error Reported.vi"("Additional Information"=w310, "Error"=w317) -> ()  [unwired: 9 in, 1 out]
    }
  }
  n200 = Merge Errors(w27, w30) -> (w26:errorcluster)
  n201 = call "Close Module.vi"("error in"=w26, "Module Admin in"=w15) -> ("error out"=w28:errorcluster, "External Launch"=w8:bool, "Module Admin out"=w9:refnum<class "Delacor_lib_QMH_Module Admin.lvclass">)  [unwired: 7 in]
  n202 = Unregister For Events(event registration refnum=w14, error in=w28) -> (error out=w25:errorcluster)
  "error out" <- w25
  n203 = case "External Launch?" shown="True" w8 {
    tunnel: w25 -> [_ w318]
    frame False {
    }
    frame True {
      n204 = case shown="No Error" w318 {
        frame No Error {
          n205 = invoke on="Invoke Node" class="VI" method="FP.Close"() -> ()  [unwired: 3 in, 3 out]
        }
        frame Error {
          n206 = disable-structure shown="Default" {
            frame condition #0 (active) {
              n207 = invoke class="VI" method="FP.Open"("Activate"=TRUE ("Activate?")) -> ()  [unwired: 4 in, 5 out]
            }
            frame condition #1 {
              # "Don't show panel on error if running inside a built EXE."
            }
          }
        }
      }
    }
  }
  n208 = local write "Module Admin"(w9) -> ()
